vi "Create Measurement.vi"(8 "error in":errorcluster, 10 "ms timeout":i32=30000) -> (0 "error out":errorcluster, 3 "gRPCid out":T1)   [LabVIEW 2021, in "MeasurementServerTests.lvlib" / "Measurement Service Tests.lvlib" / "Continuous Counting Client.lvlib"]
doc: "Create client for the measurement service and complete metadata registration."
uses:
  Continuous Counting Client.lvlib
  <vilib>/gRPC/LabVIEW gRPC Library/Shared/grpcId.ctl
  gRPC/Generated APIs/ni/measurementlink/discovery/v1/RPC Messages/ni_measurementlink_discovery_v1_ResolveServiceRequest.ctl
  controls/Measurement Results.ctl
  controls/Measurement Configuration.ctl
  <vilib>/gRPC/LabVIEW gRPC Library/grpc-lvsupport-release.lvlib
  gRPC/Generated APIs/ni/measurementlink/discovery/v1/ni.measurementlink.discovery.v1.api.lvlib
  gRPC/Generated APIs/ni/measurementlink/measurement/v2/Measurement Service Client V2/Measurement Service Client V2.lvlib
  Runtime/Clients/Discovery V1/NI Discovery V1 Client.lvlib
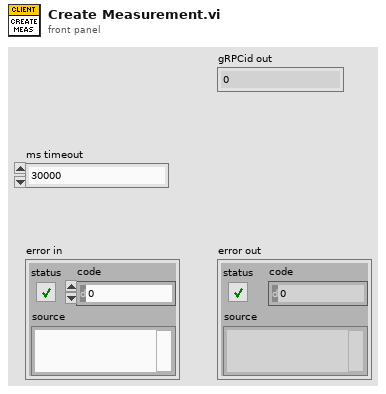
[diagram p1: front panel]
types:
  T1 = typedef "grpc-lvsupport-release.lvlib/grpcId.ctl" = u64
  T2 = typedef "MeasurementServerTests.lvlib/Measurement Service Tests.lvlib/Continuous Counting Client.lvlib/Measurement Configuration.ctl" = cluster{"ms update interval":u32}
  T3 = typedef "MeasurementServerTests.lvlib/Measurement Service Tests.lvlib/Continuous Counting Client.lvlib/Measurement Results.ctl" = cluster{"current count":i64}
  T4 = typedef "ni.measurementlink.discovery.v1.api.lvlib/ni_measurementlink_discovery_v1_ResolveServiceRequest.ctl" = cluster{"provided_interface":string, "service_class":string, "deployment_target":string, "version":string}
  T5 = typedef "ni.measurementlink.discovery.v1.api.lvlib/ni_measurementlink_discovery_v1_ServiceLocation.ctl" = cluster{"location":string, "insecure_port":string, "ssl_authenticated_port":string}
  T6 = typedef "grpc-lvsupport-release.lvlib/Enum Metadata.ctl" = cluster{"Version":i32, "Name":string, "Type Url":string, "Enum Values":string, "Allow Alias":bool}
  T7 = typedef "grpc-lvsupport-release.lvlib/Message Metadata.ctl" = cluster{"Version":i32, "Name":string, "Type Url":string, "Elements":T8[], "Has Oneof":bool}
  T8 = typedef "grpc-lvsupport-release.lvlib/Message Element Metadata.ctl" = cluster{"Field Name":string, "Embedded Message Name":string, "Protobuf Index":i32, "MessageElementType":T9, "Repeated":bool, "Is in Oneof":bool, "Oneof Container Name":string}
  T9 = typedef "grpc-lvsupport-release.lvlib/Message Element Type.ctl" = enum32{"Int32Value", "FloatValue", "DoubleValue", "BoolValue", "StringValue", "MessageValue", "Int64Value", "UInt32Value", "UInt64Value", "EnumValue", "Bytes", "Fixed64", "Fixed32", "SFixed64", "SFixed32", "SInt64", "SInt32"}
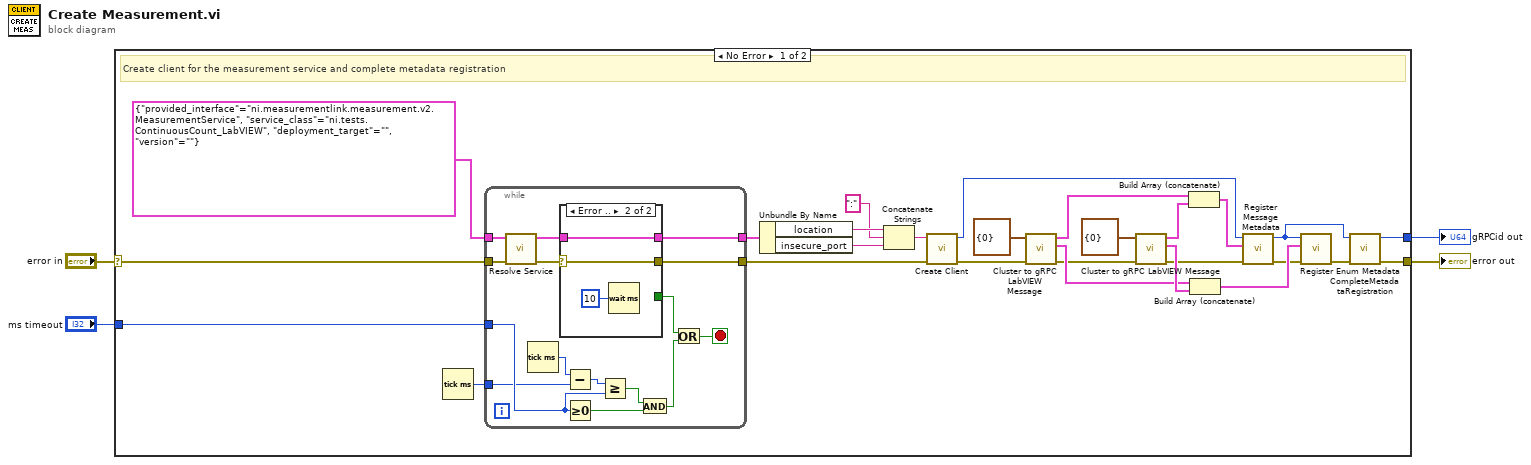
[diagram p0: block diagram]
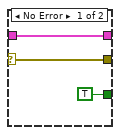
[diagram p2: hidden frame]
diagram:
  n1 = case shown="No Error" "error in" {
    selector: "error in" -> [w7 w53]
    tunnel: [w21 w53] -> w3
    tunnel: [w20 _] -> w2
    tunnel: "ms timeout" -> [w6 _]
    frame No Error {
      # "Create client for the measurement service and complete metadata registration"
      n2 = Tick Count (ms)() -> (millisecond timer value=w5:u32)
      n3 = while {
        tunnel: T4 {"provided_interface"="ni.measurementlink.measurement.v2.MeasurementService", "service_class"="ni.tests.ContinuousCount_LabVIEW", "deployment_target"="", "version"=""} ("resolve service request data") -> [w46]
        tunnel: [w42] -> w9
        tunnel: w7 -> [w45]
        tunnel: [w34] -> w8
        tunnel: w6 -> [w36]
        tunnel: w5 -> [w35]
        stop <- w33 stop-if-true
        n4 = call "Resolve Service.vi"("error in"=w45, "request data"=w46) -> ("error out"=w44:errorcluster, "response data"=w43:T5)  [unwired: 8 in]
        n5 = Tick Count (ms)() -> (millisecond timer value=w41:u32)
        n6 = case shown="Error .." w44 {
          selector: w44 -> [w49 w52]
          tunnel: [w49 w52] -> w34
          tunnel: w43 -> [w48 w51]
          tunnel: [w48 w51] -> w42
          tunnel: [TRUE ("x") _] -> w32
          frame No Error {
          }
          frame Error {
            n7 = Wait (ms)(milliseconds to wait=u32 10) -> ()  [unwired: 1 out]
          }
        }
        n8 = Subtract(x=w41, y=w35) -> (x-y=w40:u32)
        n9 = Greater Or Equal To 0?(x=w36) -> (x >= 0?=w38:bool)
        n10 = Greater Or Equal?(x=w40, y=w36) -> (x >= y?=w39:bool)
        n11 = And(x=w39, y=w38) -> (x .and. y?=w37:bool)
        n12 = Or(x=w32, y=w37) -> (x .or. y?=w33:bool)
      }
      n13 = Unbundle By Name(w9) -> ("location"=w18:string, "insecure_port"=w17:string)
      n14 = Concatenate Strings(w18, ":" ("string"), w17) -> (w11:string)
      n15 = call "Create Client.vi"("error in"=w8, "address"=w11) -> ("error out"=w13:errorcluster, "gRPC ID Out"=w12:T1)  [unwired: 8 in]
      n16 = call <vilib>:"Cluster to gRPC LabVIEW Message.vi"("error in"=w13, "Cluster"=T2 {"ms update interval"=0} ("ConfigurationParameter")) -> ("error out"=w19:errorcluster, "gRPC Enum Metadata out"=w29:T6[], "gRPC Message Metadata []"=w25:T7[])  [unwired: 7 in]
      n17 = call <vilib>:"Cluster to gRPC LabVIEW Message.vi"("error in"=w19, "Cluster"=T3 {"current count"=0} ("OutputParameter")) -> ("error out"=w22:errorcluster, "gRPC Enum Metadata out"=w30:T6[], "gRPC Message Metadata []"=w23:T7[])  [unwired: 7 in]
      n18 = Build Array (concatenate)(w25, w23) -> (w24:T7[])
      n19 = Build Array (concatenate)(w29, w30) -> (w28:T6[])
      n20 = call <vilib>:"Register Message Metadata.vi"("error in"=w22, "Messages"=w24, "gRPCid in"=w12) -> ("error out"=w26:errorcluster, "gRPCid out"=w31:T1)  [unwired: 7 in]
      n21 = call <vilib>:"Register Enum Metadata.vi"("error in"=w26, "Enum Metadata"=w28, "gRPCid in"=w31) -> ("error out"=w27:errorcluster)  [unwired: 7 in, 1 out]
      n22 = call <vilib>:"CompleteMetadataRegistration.vi"("error in"=w27, "gRPC ID in"=w31) -> ("error out"=w21:errorcluster, "gRPC ID Out"=w20:T1)  [unwired: 8 in]
    }
    frame Error {
      # "Pass"
    }
  }
  "error out" <- w3
  "gRPCid out" <- w2
